vi "Find Outputs in Dictionary.vi"(8 "error in (no error)":errorcluster, 9 "processing data dictionary":refnum<class "data dictionary.lvclass">, 10 "PID Channels In":T2(array[cluster]), 11 "Tagbus PID Module runtime in":refnum<class "Tagbus PID Module runtime.lvclass">) -> (0 "error out":errorcluster, 2 "Outputs":T1(array[cluster]), 3 "Tagbus PID Module runtime out":refnum<class "Tagbus PID Module runtime.lvclass">)   [LabVIEW 2014, in "Tagbus PID Module runtime.lvclass"]
uses:
  Tagbus PID Module runtime.lvclass
  <vilib>/NI/Tag Bus/dictionary/data dictionary.lvclass
  <vilib>/NI/Tag Bus Module Framework/channel/TBM channel.lvclass
  Tagbus PID Module runtime.lvclass/Tagbus PID Module runtime.ctl
  <vilib>/NI/Tag Bus/tag/Data Type.ctl
  <vilib>/NI/Tag Bus/tag/tag descriptor.lvclass
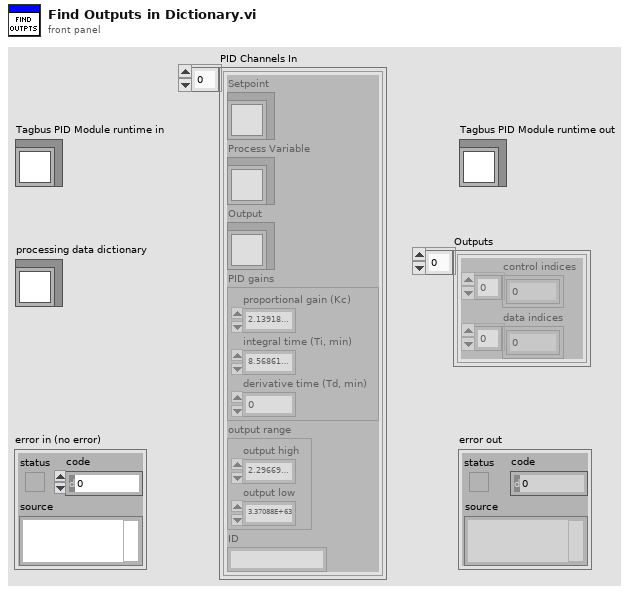
[diagram p1: front panel]
types:
  T1 = cluster{"control indices":i32[], "data indices":i32[]}[]
  T2 = cluster{"Setpoint":refnum<class "TBM channel.lvclass">, "Process Variable":refnum<class "TBM channel.lvclass">, "Output":refnum<class "TBM channel.lvclass">, "PID gains":cluster{"proportional gain (Kc)":dbl, "integral time (Ti, min)":dbl, "derivative time (Td, min)":dbl}, "output range":cluster{"output high":dbl, "output low":dbl}, "ID":string}[]
  T3 = typedef "tag bus.lvlib/tag descriptor.lvclass/Data Type.ctl" = enum16{"Double", "Single", "I64", "I32", "I16", "I8", "U64", "U32", "U16", "U8", "Boolean", "String", "Array of Double", "Array of Single", "Array of I64", "Array of I32", "Array of I16", "Array of I8", "Array of U64", "Array of U32", "Array of U16", "Array of U8", "Array of Boolean", "Array of String"}
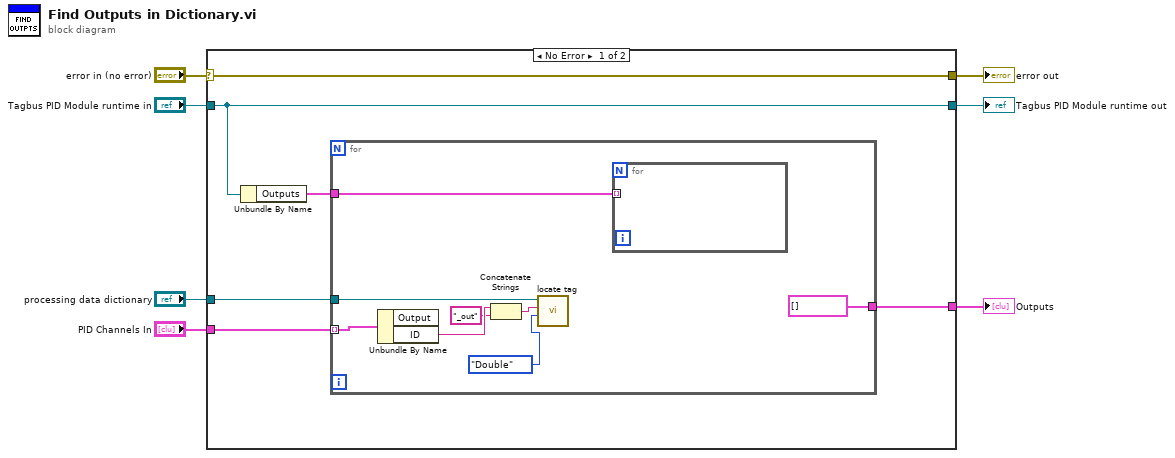
[diagram p0: block diagram]
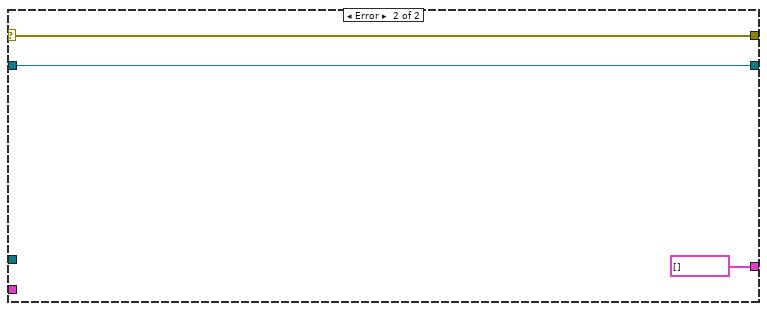
[diagram p2: hidden frame]
diagram:
  n1 = case shown="No Error" "error in (no error)" {
    selector: "error in (no error)" -> [w13 w24]
    tunnel: [w13 w24] -> w2
    tunnel: "processing data dictionary" -> [w12 _]
    tunnel: "PID Channels In" -> [w11 _]
    tunnel: "Tagbus PID Module runtime in" -> [w8 w22]
    tunnel: [w9 T1 [] ("Setpoints")] -> w1
    tunnel: [w8 w22] -> w3
    frame No Error {
      n2 = Unbundle By Name(w8) -> ("Outputs"=w10:T1)
      n3 = for {
        tunnel: w12 -> [w19]
        tunnel: w11 -> [w20] mode=indexing
        tunnel: w10 -> [w17]
        tunnel: [T1 [] ("Setpoints")] -> w9
        n4 = Unbundle By Name(w20) -> ("ID"=w15:string)  [unwired: 1 out]
        n5 = Concatenate Strings(w15, "_out" ("string")) -> (w16:string)
        n6 = call <vilib>:"locate tag.vi"("data type"=Data_Type."Double", "name"=w16, "data dictionary in"=w19) -> ()  [unwired: 6 in, 3 out]
        n7 = for {
          tunnel: w17 -> [_] mode=indexing
        }
      }
    }
    frame Error {
    }
  }
  "error out" <- w2
  "Tagbus PID Module runtime out" <- w3
  "Outputs" <- w1
